vi "Apply Label Font.vi"(7 "properties to ignore":variant, 8 "error in (no error)":errorcluster, 9 "scaling settings":T1={"scaling factor"={"horizontal"=1.0, "vertical"=1.0}, "scale text"=FALSE} {"scaling factor"."vertical" min=0.0; "scaling factor"."horizontal" min=0.0}, 10 "Ctl Refnum":refnum<vi>, 11 "Control Layout in":refnum<class "Control Layout.lvclass">) -> (0 "error out":errorcluster, 1 "applied?":bool, 3 "Control Layout out":refnum<class "Control Layout.lvclass">)   [LabVIEW 2010, in "NI_SE_Front Panel Layout.lvlib" / "Control Layout.lvclass"]
uses:
  Control Layout.lvclass
  Scaling Factor_Options.ctl
  XY Scaling Factor.ctl
  Control Layout.lvclass/Control Layout.ctl
  Properties To Ignore.vi
  NI_SE_Front Panel Layout.lvlib
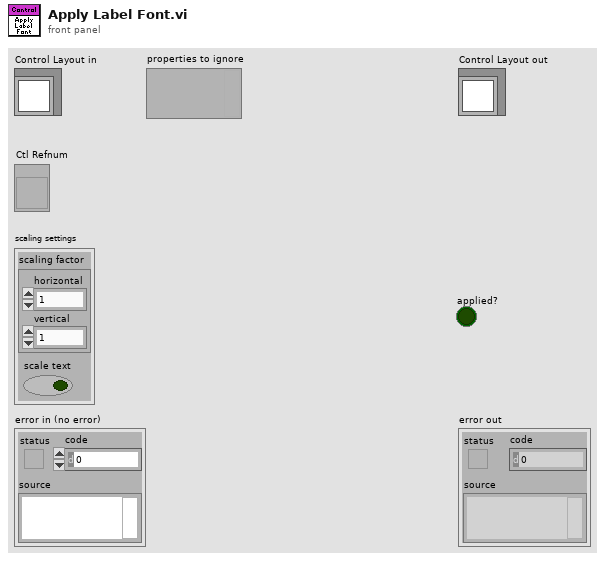
[diagram p1: front panel]
types:
  T1 = typedef "NI_SE_Front Panel Layout.lvlib/Scaling Factor_Options.ctl" = cluster{"scaling factor":T2, "scale text":bool}
  T2 = typedef "NI_SE_Front Panel Layout.lvlib/XY Scaling Factor.ctl" = cluster{"horizontal":dbl, "vertical":dbl}
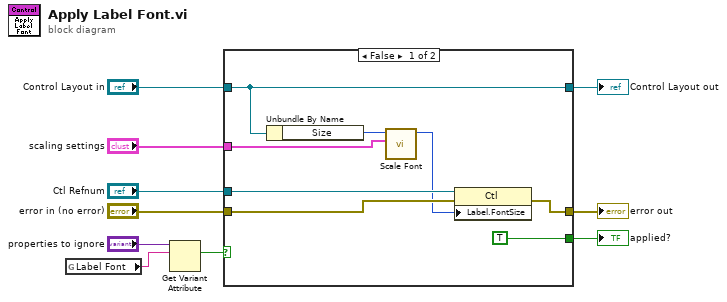
[diagram p0: block diagram]
diagram:
  n1 = global read "Properties To Ignore.vi" "Label Font"() -> (w2:string)
  n2 = Get Variant Attribute(Variant="properties to ignore", name=w2) -> (found=w4:bool)  [unwired: 2 in, 3 out]
  n3 = case shown="False" w4 {
    tunnel: "error in (no error)" -> [w18 w19]
    tunnel: [w17 w19] -> w9
    tunnel: "Control Layout in" -> [w12 w20]
    tunnel: "scaling settings" -> [w16 _]
    tunnel: "Ctl Refnum" -> [w15 _]
    tunnel: [w12 w20] -> w3
    tunnel: [TRUE _] -> w1
    frame False {
      n4 = Unbundle By Name(w12) -> ("Size"=w14:u16)
      n5 = call "Scale Font.vi"("scaling settings"=w16, "font size in"=w14) -> ("font size out"=w13:u16)  [unwired: 9 in]
      n6 = property class="Ctl"(reference=w15, error in=w18, "Label.FontSize"=w13) -> (error out=w17:errorcluster)  [unwired: 1 out]
    }
    frame True {
    }
  }
  "error out" <- w9
  "Control Layout out" <- w3
  "applied?" <- w1
